vi "FT10_Log Diff Volt LVM Values.vi"(8 "error in (no error)":errorcluster, 9 "Log Cluster in":T5, 10 "Date & Time string":string, 11 "Log Loop Cluster in":T1={"tdms file out"=refnum, "t0"="", "Generator Serial Number in"="T1234567DX"}) -> (0 "error out":errorcluster, 1 "Log Cluster out":T5, 2 "Diff Volt Wvfrm filename":string, 3 "Log Loop Cluster out":T1={"tdms file out"=refnum, "t0"="", "Generator Serial Number in"="T1234567DX"})   [LabVIEW 2015]
doc: "Saves diff voltage to LVM files each time measuremnet is taken."
uses:
  Controls/Control_Log Cluster.ctl
  Controls/Control_Log Time.ctl
  Controls/Control_Log Waveform Cluster - Current.ctl
  Controls/Control_Log Analysis Cluster - Current.ctl
  Controls/Control_Log Activation Settings Cluster.ctl
  Controls/Control_Log Unitherm Load.ctl
  Controls/Control_Log Port.ctl
  Controls/Control_Log Mode.ctl
  Controls/Control_Log Power Level.ctl
  Controls/Control_Log Waveform Cluster - Diff Voltage.ctl
  Controls/Control_Log Analysis Cluster - Diff Voltage.ctl
  Controls/Control_Log Loop Cluster.ctl
  Controls/Control_Log TDMS Filename.ctl
  Controls/Control_Log t0.ctl
  Controls/Control_Serial Number.ctl
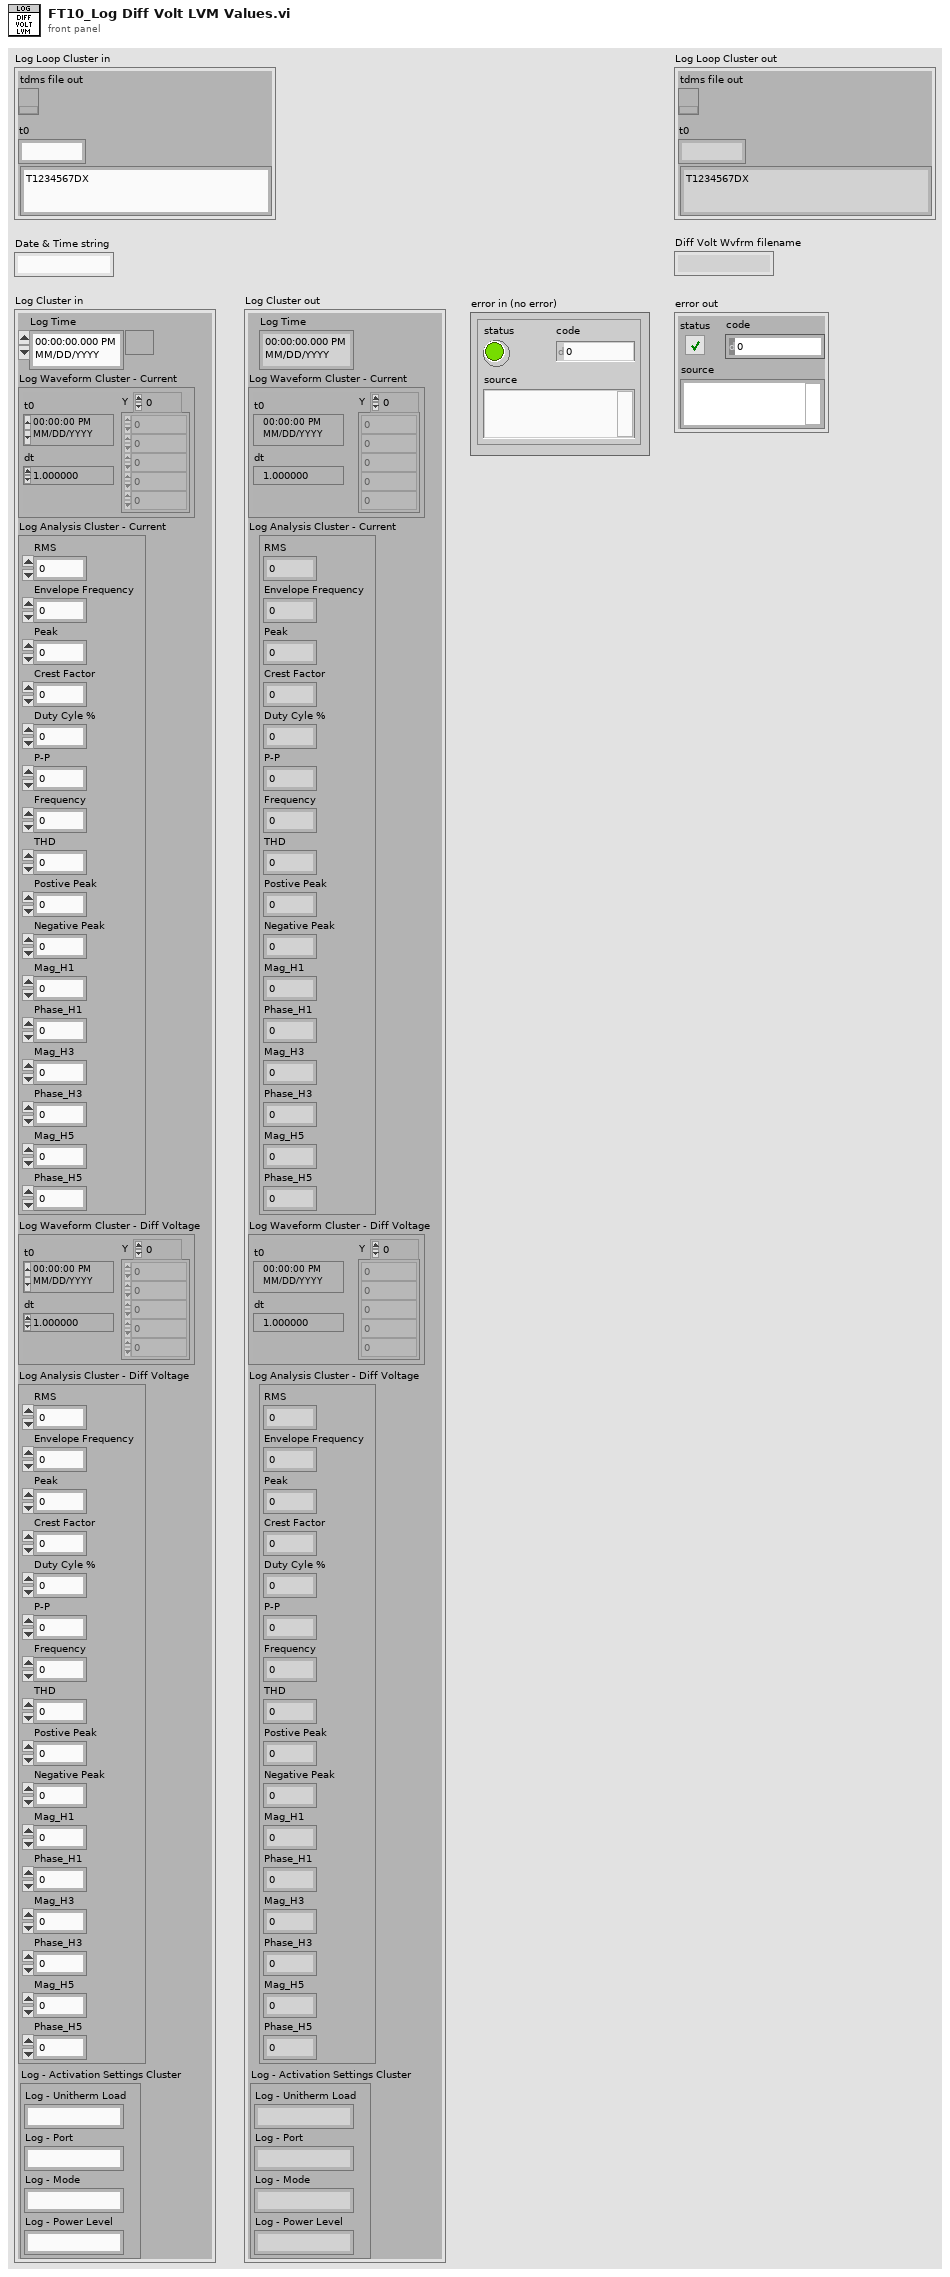
[diagram p1: front panel]
types:
  T1 = typedef "Control_Log Loop Cluster.ctl" = cluster{"tdms file out":T2, "t0":T3, "Generator Serial Number in":T4}
  T2 = typedef "Control_Log TDMS Filename.ctl" = refnum<k34>
  T3 = typedef "Control_Log t0.ctl" = string
  T4 = typedef "Control_Serial Number.ctl" = string
  T5 = typedef "Control_Log Cluster.ctl" = cluster{"Log Time":T6, "Log Waveform Cluster - Current":T7, "Log Analysis Cluster - Current":T8, "Log - Activation Settings Cluster":T9, "Log Waveform Cluster - Diff Voltage":T14, "Log Analysis Cluster - Diff Voltage":T15}
  T6 = typedef "Control_Log Time.ctl" = timestamp
  T7 = typedef "Control_Log Waveform Cluster - Current.ctl" = waveform(dbl)
  T8 = typedef "Control_Log Analysis Cluster - Current.ctl" = cluster{"RMS":dbl, "Envelope Frequency":dbl, "Peak":dbl, "Crest Factor":dbl, "Duty Cyle %":dbl, "P-P":dbl, "Frequency":dbl, "THD":dbl, "Postive Peak":dbl, "Negative Peak":dbl, "Mag_H1":dbl, "Phase_H1":dbl, "Mag_H3":dbl, "Phase_H3":dbl, "Mag_H5":dbl, "Phase_H5":dbl}
  T9 = typedef "Control_Log Activation Settings Cluster.ctl" = cluster{"Log - Unitherm Load":T10, "Log - Port":T11, "Log - Mode":T12, "Log - Power Level":T13}
  T10 = typedef "Control_Log Unitherm Load.ctl" = string
  T11 = typedef "Control_Log Port.ctl" = string
  T12 = typedef "Control_Log Mode.ctl" = string
  T13 = typedef "Control_Log Power Level.ctl" = string
  T14 = typedef "Control_Log Waveform Cluster - Diff Voltage.ctl" = waveform(dbl)
  T15 = typedef "Control_Log Analysis Cluster - Diff Voltage.ctl" = cluster{"RMS":dbl, "Envelope Frequency":dbl, "Peak":dbl, "Crest Factor":dbl, "Duty Cyle %":dbl, "P-P":dbl, "Frequency":dbl, "THD":dbl, "Postive Peak":dbl, "Negative Peak":dbl, "Mag_H1":dbl, "Phase_H1":dbl, "Mag_H3":dbl, "Phase_H3":dbl, "Mag_H5":dbl, "Phase_H5":dbl}
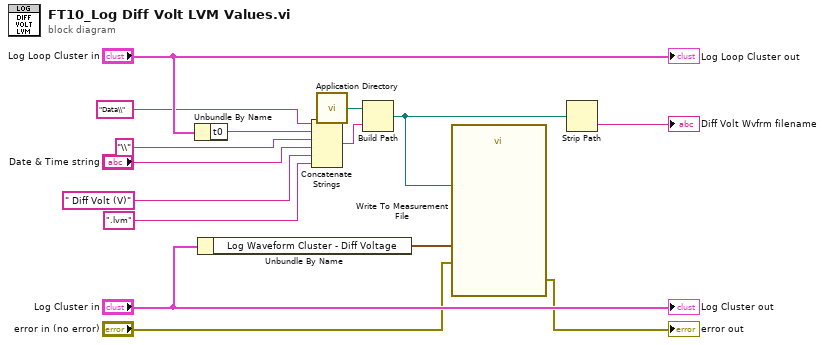
[diagram p0: block diagram]
diagram:
  n1 = Unbundle By Name("Log Loop Cluster in") -> ("t0"=w10:T3)
  n2 = Unbundle By Name("Log Cluster in") -> ("Log Waveform Cluster - Diff Voltage"=w8:T14)
  n3 = Concatenate Strings("Data\\" ("string"), w10, "\\" ("string"), "Date & Time string", " Diff Volt (V)" ("name or relative path"), ".lvm" ("string")) -> (w2:string)
  n4 = call <vilib>:"Application Directory.vi"() -> ("Application Directory"=w1:path)
  n5 = Build Path(base path=w1, name or relative path=w2) -> (appended path=w9:path)
  n6 = call "Write To Measurement File"("Signals"=w8, "error in (no error)"="error in (no error)", "Filename"=w9) -> ("error out"=→"error out":errorcluster)  [unwired: 14 in, 2 out]
  n7 = Strip Path(path=w9) -> (name=→"Diff Volt Wvfrm filename":string)  [unwired: 1 out]
  "Log Cluster out" <- "Log Cluster in"
  "Log Loop Cluster out" <- "Log Loop Cluster in"
